vi "Sqlite Query.vi"(0 "DB Path":string, 1 "SQL Query":string, 5 "Include RowID":bool, 7 "Tables Name":string, 11 "error in (no error)":errorcluster) -> (3 "Results":string[][](array[string]), 4 "DB Path Out":string, 15 "error out":errorcluster)   [LabVIEW 2016]
uses:
  <userlib>/_LVST/sqlite_api/Core/Query/SQLite_Query-Standard.vi
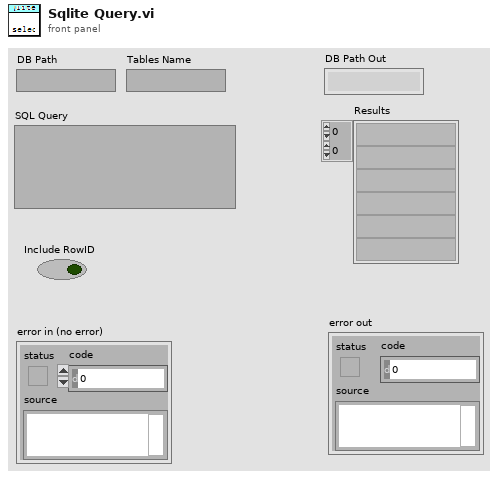
[diagram p1: front panel]
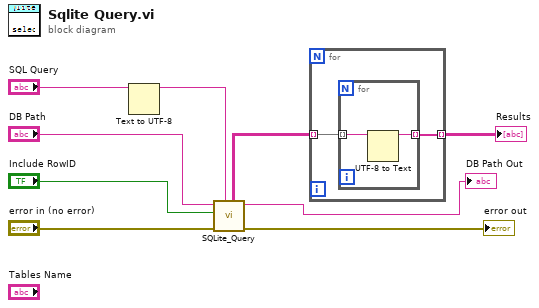
[diagram p0: block diagram]
diagram:
  n1 = Text to UTF-8(11:"SQL Query") -> (3:w4:string)  [unwired: 2 in, 1 out]
  n2 = call-poly <userlib>:"SQLite_Query.vi"("SQL Query"=w4, "error in (no error)"="error in (no error)", "Include RowID"="Include RowID", "DB Path"="DB Path") -> ("error out"=→"error out":errorcluster, "DB Path Out"=→"DB Path Out":string, "Results"=w3:string[][])  [unwired: 2 in, 1 out]
  n3 = for {
    tunnel: w3 -> [w11] mode=indexing
    tunnel: [w10] -> w9 mode=indexing
    n4 = for {
      tunnel: w11 -> [w13] mode=indexing
      tunnel: [w12] -> w10 mode=indexing
      n5 = UTF-8 to Text(11:w13) -> (3:w12:string)  [unwired: 2 in, 1 out]
    }
  }
  "Results" <- w9
